vi "Lab Panel V5.22.vi"() -> ()   [LabVIEW 2013] (continued)
            n3218 = local read "TEMP START LAB01-1"() -> (w5918:cluster{"TL":dbl, "TN":dbl})
            n3219 = local read "TEMP START LAB05-2"() -> (w5909:cluster{"TL":dbl, "TN":dbl})
            n3220 = local read "TEMP START LAB05-1"() -> (w5910:cluster{"TL":dbl, "TN":dbl})
            n3221 = local read "run lab03-2"() -> (w5977:bool)
            n3222 = local read "TEMP START LAB03-2"() -> (w5913:cluster{"TL":dbl, "TN":dbl})
            n3223 = local read "TEMP START LAB03-1"() -> (w5914:cluster{"TL":dbl, "TN":dbl})
            n3224 = local read "run lab02-1"() -> (w5980:bool)
            n3225 = local read "run lab03-1"() -> (w5978:bool)
            n3226 = local read "run lab01-2"() -> (w5981:bool)
            n3227 = local read "run lab02-2"() -> (w5979:bool)
            n3228 = local read "run lab01-1"() -> (w5982:bool)
            n3229 = global write "Global display 1.vi" "5-2 R/S"(w5973) -> ()
            n3230 = global write "Global display 1.vi" "5-1 R/S"(w5974) -> ()
            n3231 = global write "Global display 1.vi" "4-2 R/S"(w5975) -> ()
            n3232 = global write "Global display 1.vi" "4-1 R/S"(w5976) -> ()
            n3233 = global write "Global display 1.vi" "3-2 R/S"(w5977) -> ()
            n3234 = global write "Global display 1.vi" "1-2 R/S"(w5981) -> ()
            n3235 = global write "Global display 1.vi" "2-1 R/S"(w5980) -> ()
            n3236 = global write "Global display 1.vi" "3-1 R/S"(w5978) -> ()
            n3237 = global write "Global display 1.vi" "2-2 R/S"(w5979) -> ()
            n3238 = global write "Global display 1.vi" "1-1 R/S"(w5982) -> ()
            n3239 = global write "Global display 3.vi" "TEMP ST 05-2"(w5909) -> ()
            n3240 = global write "Global display 3.vi" "TEMP ST 05-1"(w5910) -> ()
            n3241 = global write "Global display 3.vi" "TEMP ST 03-2"(w5913) -> ()
            n3242 = global write "Global display 3.vi" "TEMP ST 04-2"(w5911) -> ()
            n3243 = global write "Global display 3.vi" "TEMP ST 01-1"(w5918) -> ()
            n3244 = global write "Global display 3.vi" "TEMP ST 01-2"(w5917) -> ()
            n3245 = global write "Global display 3.vi" "TEMP ST 04-1"(w5912) -> ()
            n3246 = global write "Global display 3.vi" "TEMP ST 02-1"(w5916) -> ()
            n3247 = global write "Global display 3.vi" "TEMP ST 02-2"(w5915) -> ()
            n3248 = global write "Global display 3.vi" "TEMP ST 03-1"(w5914) -> ()
            n3249 = local read "DISP LAB04-2"() -> (w5965:T4)
            n3250 = local read "DISP LAB05-1"() -> (w5964:T4)
            n3251 = local read "DISP LAB04-1"() -> (w5966:T4)
            n3252 = local read "DISP LAB05-2"() -> (w5963:T4)
            n3253 = local read "DISP LAB03-1"() -> (w5968:T4)
            n3254 = local read "DISP LAB03-2"() -> (w5967:T4)
            n3255 = local read "DISP LAB01-2"() -> (w5971:T4)
            n3256 = local read "DISP LAB02-1"() -> (w5970:T4)
            n3257 = local read "DISP LAB02-2"() -> (w5969:T4)
            n3258 = local read "DISP LAB01-1"() -> (w5972:T4)
            n3259 = local read "TEMP RISE LAB05-1"() -> (w5900:cluster{"TL":dbl, "TN":dbl})
            n3260 = local read "TEMP RISE LAB05-2"() -> (w5899:cluster{"TL":dbl, "TN":dbl})
            n3261 = local read "TEMP RISE LAB04-2"() -> (w5901:cluster{"TL":dbl, "TN":dbl})
            n3262 = local read "TEMP RISE LAB04-1"() -> (w5902:cluster{"TL":dbl, "TN":dbl})
            n3263 = local read "TEMP RISE LAB03-2"() -> (w5903:cluster{"TL":dbl, "TN":dbl})
            n3264 = local read "TEMP RISE LAB03-1"() -> (w5904:cluster{"TL":dbl, "TN":dbl})
            n3265 = local read "TEMP RISE LAB01-2"() -> (w5907:cluster{"TL":dbl, "TN":dbl})
            n3266 = local read "TEMP RISE LAB02-2"() -> (w5905:cluster{"TL":dbl, "TN":dbl})
            n3267 = local read "TEMP RISE LAB01-1"() -> (w5908:cluster{"TL":dbl, "TN":dbl})
            n3268 = local read "TEMP RISE LAB02-1"() -> (w5906:cluster{"TL":dbl, "TN":dbl})
            n3269 = global write "Global display 2.vi" "DISP LAB05-1"(w5964) -> ()
            n3270 = global write "Global display 2.vi" "DISP LAB05-2"(w5963) -> ()
            n3271 = global write "Global display 2.vi" "DISP LAB04-2"(w5965) -> ()
            n3272 = global write "Global display 2.vi" "DISP LAB02-1"(w5970) -> ()
            n3273 = global write "Global display 2.vi" "DISP LAB02-2"(w5969) -> ()
            n3274 = global write "Global display 2.vi" "DISP LAB04-1"(w5966) -> ()
            n3275 = global write "Global display 2.vi" "DISP LAB01-2"(w5971) -> ()
            n3276 = global write "Global display 2.vi" "DISP LAB01-1"(w5972) -> ()
            n3277 = global write "Global display 2.vi" "DISP LAB03-1"(w5968) -> ()
            n3278 = global write "Global display 2.vi" "DISP LAB03-2"(w5967) -> ()
            n3279 = global write "Global display 3.vi" "TEMP RS 05-2"(w5899) -> ()
            n3280 = global write "Global display 3.vi" "TEMP RS 05-1"(w5900) -> ()
            n3281 = global write "Global display 3.vi" "TEMP RS 03-2"(w5903) -> ()
            n3282 = global write "Global display 3.vi" "TEMP RS 02-1"(w5906) -> ()
            n3283 = global write "Global display 3.vi" "TEMP RS 02-2"(w5905) -> ()
            n3284 = global write "Global display 3.vi" "TEMP RS 04-2"(w5901) -> ()
            n3285 = global write "Global display 3.vi" "TEMP RS 01-2"(w5907) -> ()
            n3286 = global write "Global display 3.vi" "TEMP RS 03-1"(w5904) -> ()
            n3287 = global write "Global display 3.vi" "TEMP RS 04-1"(w5902) -> ()
            n3288 = global write "Global display 3.vi" "TEMP RS 01-1"(w5908) -> ()
            n3289 = local read "SET LAB05-2"() -> (w5953:T5)
            n3290 = local read "SET LAB05-1"() -> (w5954:T5)
            n3291 = local read "SET LAB04-1"() -> (w5956:T5)
            n3292 = local read "SET LAB04-2"() -> (w5955:T5)
            n3293 = local read "SET LAB03-1"() -> (w5958:T5)
            n3294 = local read "SET LAB03-2"() -> (w5957:T5)
            n3295 = local read "SET LAB02-2"() -> (w5959:T5)
            n3296 = local read "SET LAB01-2"() -> (w5961:T5)
            n3297 = local read "SET LAB02-1"() -> (w5960:T5)
            n3298 = local read "SET LAB01-1"() -> (w5962:T5)
            n3299 = global write "Global display 2.vi" "SET LAB05-2"(w5953) -> ()
            n3300 = global write "Global display 2.vi" "SET LAB05-1"(w5954) -> ()
            n3301 = global write "Global display 2.vi" "SET LAB04-1"(w5956) -> ()
            n3302 = global write "Global display 2.vi" "SET LAB04-2"(w5955) -> ()
            n3303 = global write "Global display 2.vi" "SET LAB03-2"(w5957) -> ()
            n3304 = global write "Global display 2.vi" "SET LAB02-2"(w5959) -> ()
            n3305 = global write "Global display 2.vi" "SET LAB03-1"(w5958) -> ()
            n3306 = global write "Global display 2.vi" "SET LAB01-2"(w5961) -> ()
            n3307 = global write "Global display 2.vi" "SET LAB01-1"(w5962) -> ()
            n3308 = global write "Global display 2.vi" "SET LAB02-1"(w5960) -> ()
            n3309 = local read "RESULT LAB01-1"() -> (w5952:bool)
            n3310 = local read "RESULT LAB03-2"() -> (w5947:bool)
            n3311 = local read "RESULT LAB04-1"() -> (w5946:bool)
            n3312 = local read "RESULT LAB04-2"() -> (w5945:bool)
            n3313 = local read "RESULT LAB02-2"() -> (w5949:bool)
            n3314 = local read "RESULT LAB01-2"() -> (w5951:bool)
            n3315 = local read "RESULT LAB02-1"() -> (w5950:bool)
            n3316 = local read "RESULT LAB03-1"() -> (w5948:bool)
            n3317 = local read "RESULT LAB05-1"() -> (w5944:bool)
            n3318 = local read "RESULT LAB05-2"() -> (w5943:bool)
            n3319 = global write "Global display 2.vi" "RESULT LAB05-1"(w5944) -> ()
            n3320 = global write "Global display 2.vi" "RESULT LAB01-2"(w5951) -> ()
            n3321 = global write "Global display 2.vi" "RESULT LAB03-2"(w5947) -> ()
            n3322 = global write "Global display 2.vi" "RESULT LAB04-1"(w5946) -> ()
            n3323 = global write "Global display 2.vi" "RESULT LAB04-2"(w5945) -> ()
            n3324 = global write "Global display 2.vi" "RESULT LAB05-2"(w5943) -> ()
            n3325 = global write "Global display 2.vi" "RESULT LAB03-1"(w5948) -> ()
            n3326 = global write "Global display 2.vi" "RESULT LAB02-1"(w5950) -> ()
            n3327 = global write "Global display 2.vi" "RESULT LAB02-2"(w5949) -> ()
            n3328 = global write "Global display 2.vi" "RESULT LAB01-1"(w5952) -> ()
          }
          frame #21 {
            # "simulate values"
            n3329 = global write "Global display 4.vi" "LAB deg C"("LAB deg C") -> ()
          }
          frame #22 {
            # "end main and display program"
            n3330 = stacked-sequence {
              seq-local: [_ w5997 _] -> [_ _ w6000]
              tunnel: w5994 -> [w5995 _ _]
              frame #0 {
                n3331 = case shown="True" w5995 {
                  frame False {
                  }
                  frame True {
                    n3332 = One Button Dialog(message="Excessive number of USB \nresets done, re-start program.") -> ()  [unwired: 1 in, 1 out]
                  }
                }
              }
              frame #1 {
                # "check for reset error"
                n3333 = local read "Reset Error"() -> (w5997:bool)
                n3334 = case shown="True" w5997 {
                  frame False {
                  }
                  frame True {
                    n3335 = One Button Dialog(message="USB Reset ERROR, program will be stopped.\nClose program, close windows, switch panel off\nand re power panel. If error persists seek help.") -> ()  [unwired: 1 in, 1 out]
                  }
                }
              }
              frame #2 {
                # "end labview session"
                n3336 = Or(x=w6000, y="stop all") -> (x .or. y?=w5999:bool)
                n3337 = Quit LabVIEW(quit? (T)=w5999) -> ()
                n3338 = global write "Global display 1.vi" "stop disp"(w5999) -> ()
              }
            }
          }
        }
        n3339 = node-c288() -> ()  [unwired: 1 in, 1 out]
        "loops" <- w318
      }
      n3340 = node-c288(w291) -> ()  [unwired: 1 out]
    }
  }
